vi "MonoSpec50 PulseGen.vi"(5 "Abort Ref":refnum<vi>, 7 "error in":errorcluster, 8 "Moving Ref":refnum<vi>, 9 "nb pulse":i32=1000, 10 "Directions":bool=TRUE caption="Direction") -> (0 "error out":errorcluster, 3 "Aborted":bool)   [LabVIEW 2019]
doc: "Ce Vi commande la carte d'acquisition NI PCI-6052E à régler le bit de contrôle de direction et à envoyer le nombre d'impulsion voulue. Les voie de sortie utilisés pour la direction et les impulsions sont prédéterminées dans l'assistant \"Motion and Automation explorer\" (MAX)"
uses:
  <vilib>/DAQmx/write.llb/DAQmx Write (Digital Bool 1Line 1Point).vi
  <vilib>/DAQmx/miscellaneous.llb/DAQmx Fill In Error Info.vi
  <vilib>/DAQmx/configure/timing.llb/DAQmx Timing (Implicit).vi
  <resource>/objmgr/daqmx.rc
panel:
  in  "Abort":bool
  out "Moving":bool caption="Déplacement\nen cours"
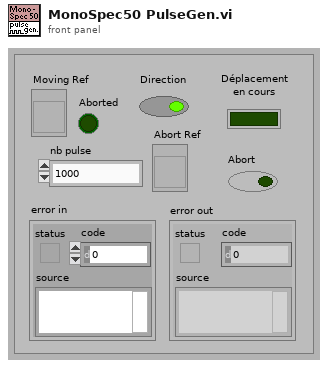
[diagram p1: front panel]
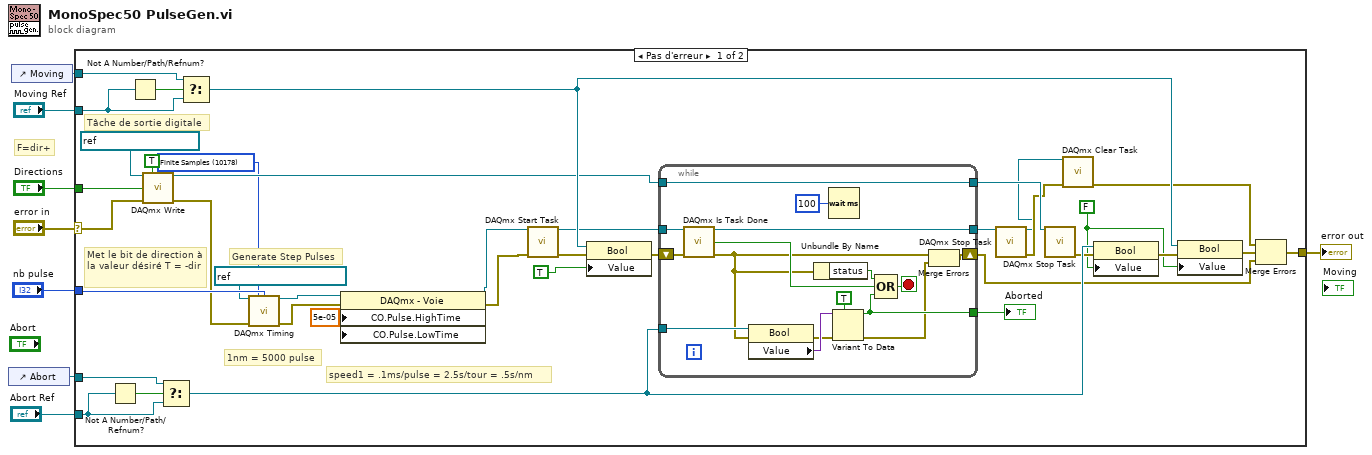
[diagram p0: block diagram]
diagram:
  # "F=dir+"
  n1 = control-ref of="Abort"() -> (w1:refnum<vi>)
  n2 = control-ref of="Moving"() -> (w3:refnum<vi>)
  n3 = case shown="Pas d'erreur" "error in" {
    selector: "error in" -> [w44 w63]
    tunnel: "nb pulse" -> [w37 _]
    tunnel: [w22 w63] -> w7
    tunnel: "Directions" -> [w45 _]
    tunnel: "Moving Ref" -> [w41 _]
    tunnel: w3 -> [w38 _]
    tunnel: "Abort Ref" -> [w30 _]
    tunnel: w1 -> [w29 _]
    frame No Error {
      w13 = 10178 items=["Finite Samples"=10178, "Continuous Samples"=10123, "Hardware Timed Single Point"=12522] ("sample mode")
      w16 = 5e-05 ("CO.Pulse.HighTime")
      w23 = FALSE ("Value")
      # "speed1 = .1ms/pulse = 2.5s/tour = .5s/nm"
      # "Generate Step Pulses"
      # "1nm = 5000 pulse"
      # "Met le bit de direction à la valeur désiré T = -dir"
      # "Tâche de sortie digitale"
      n4 = Not A Number/Path/Refnum?(number/path/refnum=w30) -> (NaN/Path/Refnum?=w31:bool)
      n5 = Not A Number/Path/Refnum?(number/path/refnum=w41) -> (NaN/Path/Refnum?=w42:bool)
      n6 = call-poly <vilib>:"DAQmx Write.vi"("task/channels in"=refnum<k21> "Direction Spectro", "auto start"=TRUE, "data"=w45, "error in"=w44) -> ("task out"=w14:refnum<k21>, "error out"=w34:errorcluster)  [unwired: 9 in, 1 out]
      n7 = Select(t=w29, s=w31, f=w30) -> (s? t:f=w26:refnum<vi>)
      n8 = Select(t=w38, s=w42, f=w41) -> (s? t:f=w39:refnum<vi>)
      n9 = call-poly <vilib>:"DAQmx Timing.vi"("task/channels in"=refnum<k21> "Sortie Pulse Spectro", "sample mode"=w13, "samples per channel"=w37, "error in"=w34) -> ("task out"=w20:refnum<k21>, "error out"=w19:errorcluster)  [unwired: 10 in]
      n10 = property class="DAQmx - Voie"(reference=w20, error in=w19, "CO.Pulse.HighTime"=w16, "CO.Pulse.LowTime"=w16) -> (reference out=w18:refnum<k21>, error out=w17:errorcluster)
      n11 = call <vilib>:"DAQmx Start Task.vi"("task/channels in"=w18, "error in"=w17) -> ("task out"=w33:refnum<k21>, "error out"=w36:errorcluster)  [unwired: 12 in]
      n12 = property class="Bool"(reference=w39, error in=w36, "Value"=TRUE) -> (error out=w40:errorcluster)  [unwired: 1 out]
      n13 = while {
        shift-right: [w54] -> w21
        shift-left: w40 -> [w57]
        tunnel: [w60] -> w12
        tunnel: w33 -> [w56]
        tunnel: w26 -> [w53]
        tunnel: [w49] -> w27
        tunnel: [w47] -> w15
        tunnel: w14 -> [w47]
        stop <- w62 stop-if-true
        n14 = call <vilib>:"DAQmx Is Task Done.vi"("task/channels in"=w56, "error in"=w57) -> ("task out"=w60:refnum<k21>, "task done?"=w59:bool, "error out"=w52:errorcluster)  [unwired: 11 in]
        n15 = property class="Bool"(reference=w53, error in=w52) -> (error out=w50:errorcluster, "Value"=w51:variant)  [unwired: 1 out]
        n16 = Unbundle By Name(w52) -> ("status"=w61:bool)
        n17 = Wait (ms)(milliseconds to wait=u32 100) -> ()  [unwired: 1 out]
        n18 = Variant To Data(error in=w50, type=TRUE ("Value"), Variant=w51) -> (data=w49:bool, error out=w48:errorcluster)
        n19 = Compound Arithmetic op=OR(w61, w59, w49) -> (w62:bool)
        n20 = Merge Errors(w52, w48) -> (w54:errorcluster)
      }
      "Aborted" <- w27
      n21 = call <vilib>:"DAQmx Stop Task.vi"("task/channels in"=w12) -> ("task out"=w10:refnum<k21>, "error out"=w11:errorcluster)  [unwired: 13 in]
      n22 = call <vilib>:"DAQmx Stop Task.vi"("task/channels in"=w15) -> ("error out"=w25:errorcluster)  [unwired: 13 in, 1 out]
      n23 = call <vilib>:"DAQmx Clear Task.vi"("task in"=w10, "error in"=w11) -> ("error out"=w9:errorcluster)  [unwired: 13 in]
      n24 = property class="Bool"(reference=w26, error in=w25, "Value"=w23) -> (error out=w24:errorcluster)  [unwired: 1 out]
      n25 = property class="Bool"(reference=w39, error in=w24, "Value"=w23) -> (error out=w32:errorcluster)  [unwired: 1 out]
      n26 = Merge Errors(w9, w32, w21) -> (w22:errorcluster)
    }
    frame Error {
    }
  }
  "error out" <- w7
